vi "OAT Resample Waveform.vi"   [LabVIEW 2017]
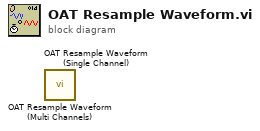
[diagram p0: block diagram]
diagram:
  n1 = call <vilib>:"OAT Resample Waveform (Multi Channels).vi"() -> ()  [unwired: 8 in, 4 out]
  n2 = call <vilib>:"OAT Resample Waveform (Single Channel).vi"() -> ()  [unwired: 8 in, 4 out]
